vi "Write State.vi"(8 "error in (no error)":errorcluster, 10 "Set":T1, 11 "SciShutt in":refnum<class "SciShutt.lvclass">) -> (0 "error out":errorcluster, 3 "SciShutt out":refnum<class "SciShutt.lvclass">)   [LabVIEW 2016, in "SciShutt.lvclass"]
uses:
  SciShutt.lvclass
  Controls/Shutter States.ctl
  BiStable/BiStableShutter.lvclass
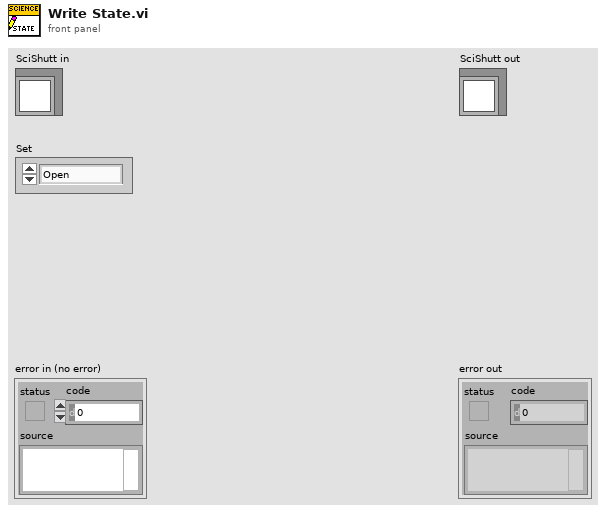
[diagram p1: front panel]
types:
  T1 = typedef "Shutter States.ctl" = enum16{"Open", "Close", "Wait", "Off", "Arm", "Idle"}
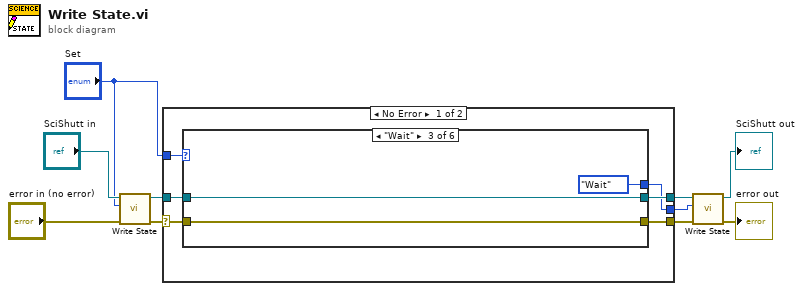
[diagram p0: block diagram]
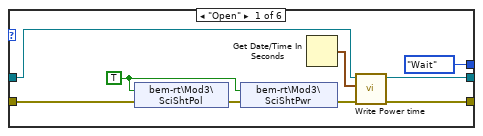
[diagram p2: hidden frame]
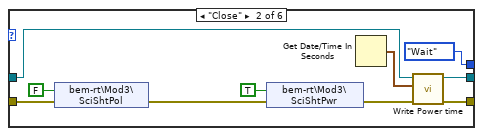
[diagram p3: hidden frame]
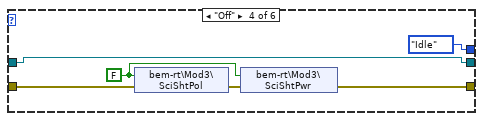
[diagram p4: hidden frame]
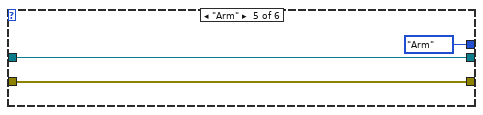
[diagram p5: hidden frame]
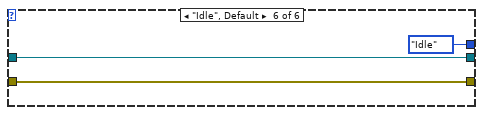
[diagram p6: hidden frame]
diagram:
  n1 = call-parent "Write State.vi"("error in (no error)"="error in (no error)", "Set"="Set", "Shutter in"="SciShutt in") -> ("error out"=w7:errorcluster, "Shutter out"=w6:refnum<class "SciShutt.lvclass">)  [unwired: 7 in]
  n2 = case shown="No Error" w7 {
    selector: w7 -> [w13 w53]
    tunnel: "Set" -> [w16 w52]
    tunnel: [w11 w53] -> w2
    tunnel: [w15 w51] -> w4
    tunnel: [w14 w52] -> w3
    tunnel: w6 -> [w12 w51]
    frame No Error {
      n3 = case shown="\"Wait\"" w16 {
        tunnel: w13 -> [w25 w33 w36 w42 w45 w48]
        tunnel: w12 -> [w18 w30 w38 w40 w47 w50]
        tunnel: [w19 w29 w38 w40 w47 w50] -> w15
        tunnel: [Shutter_States."Wait" ("Set") Shutter_States."Wait" ("Set") Shutter_States."Wait" ("Set") Shutter_States."Idle" ("Set") Shutter_States."Arm" ("Set") Shutter_States."Idle" ("Set")] -> w14
        tunnel: [w20 w28 w36 w39 w45 w48] -> w11
        frame "Open" {
          w22 = TRUE ("ExtFltSht")
          n4 = shared-variable "bem-rt\\Mod3\\SciShtPol"(w22, error in=w25) -> (error out=w23:errorcluster)
          n5 = shared-variable "bem-rt\\Mod3\\SciShtPwr"(w22, error in=w23) -> (error out=w21:errorcluster)
          n6 = Get Date/Time In Seconds() -> (seconds since 1Jan1904=w17:timestamp)
          n7 = call-dynamic "Write Power time.vi"("error in (no error)"=w21, "Power time"=w17, "BiStableShutter in"=w18) -> ("error out"=w20:errorcluster, "BiStableShutter out"=w19:refnum<class "SciShutt.lvclass">)  [unwired: 7 in]
        }
        frame "Close" {
          n8 = shared-variable "bem-rt\\Mod3\\SciShtPol"(FALSE ("SciShtPol"), error in=w33) -> (error out=w34:errorcluster)
          n9 = shared-variable "bem-rt\\Mod3\\SciShtPwr"(TRUE ("SciShtPwr"), error in=w34) -> (error out=w27:errorcluster)
          n10 = Get Date/Time In Seconds() -> (seconds since 1Jan1904=w26:timestamp)
          n11 = call-dynamic "Write Power time.vi"("error in (no error)"=w27, "Power time"=w26, "BiStableShutter in"=w30) -> ("error out"=w28:errorcluster, "BiStableShutter out"=w29:refnum<class "SciShutt.lvclass">)  [unwired: 7 in]
        }
        frame "Wait" {
        }
        frame "Off" {
          w41 = FALSE ("SciShtPol")
          n12 = shared-variable "bem-rt\\Mod3\\SciShtPol"(w41, error in=w42) -> (error out=w43:errorcluster)
          n13 = shared-variable "bem-rt\\Mod3\\SciShtPwr"(w41, error in=w43) -> (error out=w39:errorcluster)
        }
        frame "Arm" {
        }
        frame "Idle", Default {
        }
      }
    }
    frame Error {
    }
  }
  n14 = call-parent "Write State.vi"("error in (no error)"=w2, "Set"=w3, "Shutter in"=w4) -> ("error out"=→"error out":errorcluster, "Shutter out"=→"SciShutt out":refnum<class "SciShutt.lvclass">)  [unwired: 7 in]
